vi "Start_WatchDog.vi"(8 "error in (no error)":errorcluster, 10 "Caller":refnum<queue>, 11 "ModToWatch":refnum<class "Module.lvclass">) -> (0 "error out":errorcluster)   [LabVIEW 2024, in "Watchdog.lvclass"]
uses:
  Watchdog.lvclass
  Watchdog.lvclass/Watchdog.ctl
  C:/Git/JA/JQMH/RQMHCore/ModuleCore/Module.lvclass
  C:/Git/JA/JQMH/RQMHCore/Watchdog/Watchdog.lvclass
  ModuleCore/Module.lvclass
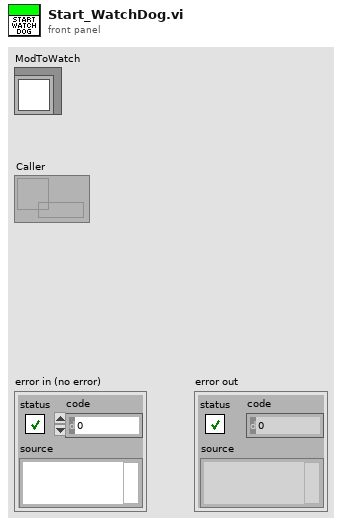
[diagram p1: front panel]
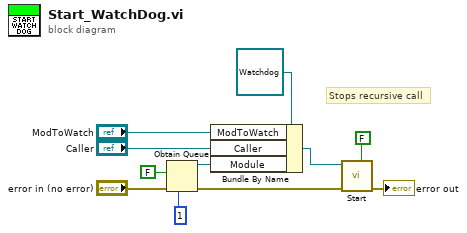
[diagram p0: block diagram]
diagram:
  # "Stops recursive call"
  n1 = Obtain Queue(max queue size (-1, unlimited)=1, element data type=FALSE, error in (no error)="error in (no error)") -> (queue out=w6:refnum<queue>, error out=w4:errorcluster)  [unwired: 2 in, 1 out]
  n2 = Bundle By Name(cluster=refnum<class "Watchdog.lvclass"> refnum ("Watchdog.lvclass"), "ModToWatch"="ModToWatch", "Caller"="Caller", "Module"=w6) -> (w9:refnum<class "Watchdog.lvclass">)
  n3 = call "Start.vi"("Autoshutdown? (T)"=FALSE, "error in (no error)"=w4, "JQMHCore in"=w9) -> ("error out"=→"error out":errorcluster)  [unwired: 6 in, 2 out]
